vi "preapre new status entry.vi"(8 "error in (no error)":errorcluster, 10 "new content":string, 11 "module id":i32) -> (0 "error out":errorcluster, 3 "new entry":string)   [LabVIEW 2024, in "status manager.lvlib"]
uses:
  status manager.lvlib
  <vilib>/Utility/error.llb/DialogType.ctl
  <vilib>/Hampel Software Engineering/HSE Logger/hse-logger.lvlib
  <vilib>/Hampel Software Engineering/Git API/Git API/GIT-api.lvclass
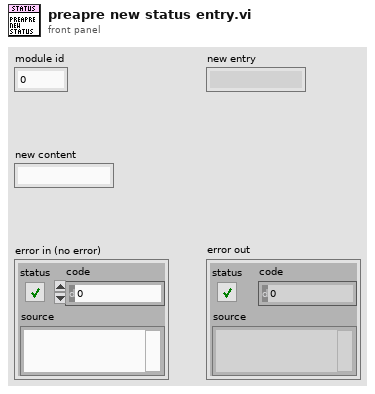
[diagram p1: front panel]
types:
  T1 = typedef "DialogType.ctl" = u16
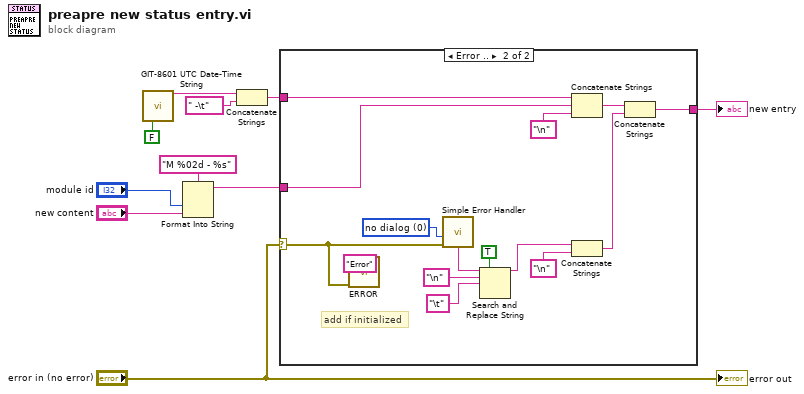
[diagram p0: block diagram]
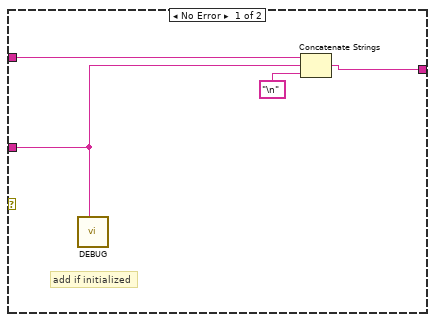
[diagram p2: hidden frame]
diagram:
  n1 = call <vilib>:"GIT-8601 UTC Date-Time String.vi"("Include TZ? (T)"=FALSE) -> ("8601 Date/Time String"=w8:string)  [unwired: 12 in, 2 out]
  n2 = Format Into String(format string="M %02d - %s", "module id", "new content") -> (resulting string=w7:string)  [unwired: 2 in, 1 out]
  n3 = Concatenate Strings(w8, " -\t") -> (w3:string)
  n4 = case shown="Error .." "error in (no error)" {
    selector: "error in (no error)" -> [_ w18]
    tunnel: w7 -> [w11 w28]
    tunnel: [w12 w22] -> w4
    tunnel: w3 -> [w13 w23]
    frame No Error {
      # "add if initialized"
      n5 = call <vilib>:"DEBUG.vi"("Message"=w11) -> ()  [unwired: 10 in, 1 out]
      n6 = Concatenate Strings(w13, w11, "\n") -> (w12:string)
    }
    frame Error {
      w17 = T1 0 items=["no dialog", "OK message", "continue or stop message", "OK message + warnings", "continue/stop + warnings"]
      # "add if initialized"
      n7 = call <vilib>:"ERROR.vi"("Message"="Error", "error in"=w18) -> ()  [unwired: 9 in, 1 out]
      n8 = call <vilib>:"Simple Error Handler.vi"("type of dialog (OK msg:1)"=w17, "error in (no error)"=w18) -> ("message"=w16:string)  [unwired: 3 in, 4 out]
      n9 = Search and Replace String(replace all?=TRUE, input string=w16, search string="\n", replace string="\t") -> (result string=w15:string)  [unwired: 4 in, 3 out]
      n10 = Concatenate Strings(w23, w28, "\n") -> (w25:string)
      n11 = Concatenate Strings(w15, "\n") -> (w21:string)
      n12 = Concatenate Strings(w25, w21) -> (w22:string)
    }
  }
  "new entry" <- w4
  "error out" <- "error in (no error)"
